vi "Associated Power Technologies 8500 Series Step Mode.vi"() -> ()   [LabVIEW 2014]
doc: "This VI is an example for controlling the power source, APT-8500 series, of Associated Power Technologies. \n\nThis vi shows how to configure and control the APT8500 series in step mode."
uses:
  <instrlib>/Associated Power Technologies 8500 Series/Public/Configure/Step Mode/Step Mode - Add File.vi
  <instrlib>/Associated Power Technologies 8500 Series/Public/Configure/Step Mode/Step Mode - Edit File.vi
  <instrlib>/Associated Power Technologies 8500 Series/Public/Configure/Step Mode/Step Mode - Configure Step Count.vi
  <instrlib>/Associated Power Technologies 8500 Series/Public/Configure/Step Mode/Step Mode - Configure Trigger Source.vi
  <instrlib>/Associated Power Technologies 8500 Series/Public/Configure/Step Mode/Step Mode - Configure Base.vi
  <instrlib>/Associated Power Technologies 8500 Series/Public/Configure/Step Mode/Step Mode - Configure Range.vi
  <instrlib>/Associated Power Technologies 8500 Series/Public/Configure/Step Mode/Step Mode - Configure Output Waveform.vi
  <instrlib>/Associated Power Technologies 8500 Series/Public/Configure/Step Mode/Step Mode - Configure Start Angle.vi
  <instrlib>/Associated Power Technologies 8500 Series/Public/Configure/Step Mode/Step Mode - Configure AC Voltage.vi
  <instrlib>/Associated Power Technologies 8500 Series/Public/Configure/Step Mode/Step Mode - Configure Frequency.vi
  <instrlib>/Associated Power Technologies 8500 Series/Public/Configure/Step Mode/Step Mode - Configure DC Voltage.vi
  <instrlib>/Associated Power Technologies 8500 Series/Public/Configure/Step Mode/Step Mode - Configure delta AC Voltage.vi
  <instrlib>/Associated Power Technologies 8500 Series/Public/Configure/Step Mode/Step Mode - Configure delta Frequency.vi
  <instrlib>/Associated Power Technologies 8500 Series/Public/Configure/Step Mode/Step Mode - Configure delta DC Voltage.vi
  <instrlib>/Associated Power Technologies 8500 Series/Public/Configure/Step Mode/Step Mode - Configure Cycle.vi
  <instrlib>/Associated Power Technologies 8500 Series/Public/Configure/Step Mode/Step Mode - Configure Time Unit.vi
  <instrlib>/Associated Power Technologies 8500 Series/Public/Configure/Step Mode/Step Mode - Configure Dwell Time.vi
  <instrlib>/Associated Power Technologies 8500 Series/Public/Configure/Step Mode/Step Mode - Configure THD.vi
  <instrlib>/Associated Power Technologies 8500 Series/Public/Configure/Step Mode/Step Mode - Load File.vi
  <instrlib>/Associated Power Technologies 8500 Series/Public/Data/Measurement/Read All Measurements.vi
  <instrlib>/Associated Power Technologies 8500 Series/Associated Power Technologies 8500 Series.lvlib
panel:
  out "All Measurements":T1
  in  "Stop":bool
  in  "Step Mode Configurations":T2={"Step Count"=5, "Trigger Source"=0, "Base"=0, "Range"=0, "Waveform Type"=0, "Start Angle"=90, "AC Voltage"=50.0, "Frequency"=60.0, "DC Voltage"=10.0, "Delta AC Voltage"=20.0, "Delta Frequency"=10.0, "Delta DC Voltage"=10.0, "Unit"=1, "Dwell Time"=2.0, "Cycles"=2, "THD"=30.0} {"Step Count" max=50000; "Trigger Source" items=["AUTO", "MANUAL"]; "Base" items=["TIME", "CYCLE"]; "Range" items=["AUTO", "HIGH", "LOW"]; "Waveform Type" items=["Sine", "Triangle", "Square", "Clipped"]; "Start Angle" max=359; "AC Voltage" min=0.0 max=310.0; "Frequency" min=5.0 max=1200.0; "DC Voltage" min=0.0 max=420.0; "Delta AC Voltage" min=0.0 max=310.0; "Delta Frequency" min=0.0 max=1200.0; "Delta DC Voltage" min=0.0 max=420.0; "Unit" items=["MS", "SECOND", "MINUTE", "HOUR"]; "Dwell Time" min=1.0 max=999.9 step=0.1; "Cycles" max=50000; "THD" min=0.0 max=46.0 step=0.1}
  in  "Serial Configuration":T3={"Baud Rate"=115200, "Parity"=0, "Data Bits"=8, "Stop Bits"=10, "Flow Control"=0} {"Flow Control" items=["None", "XON/XOFF", "RTS/CTS", "XON/XOFF & RTS/CTS", "DTR/DSR", "XON/XOFF & DTR/DSR"]; "Stop Bits" items=["1.0"=10, "1.5"=15, "2.0"=20]; "Data Bits" items=["7"=7, "8"=8]; "Parity" items=["None", "Odd", "Even", "Mark", "Space"]; "Baud Rate" items=["300"=300, "600"=600, "1200"=1200, "2400"=2400, "4800"=4800, "9600"=9600, "19200"=19200, "38400"=38400, "115200"=115200]}
  in  "VISA resource name":refnum<visa-resource-name>
  # "Step Mode Operation of APT-8500 Series"
  # "Initialization"
  # "Configurations"
  # "Meters"
  # "(c) 2020 Associated Power Technologies.  ALL RIGHTS RESERVED."
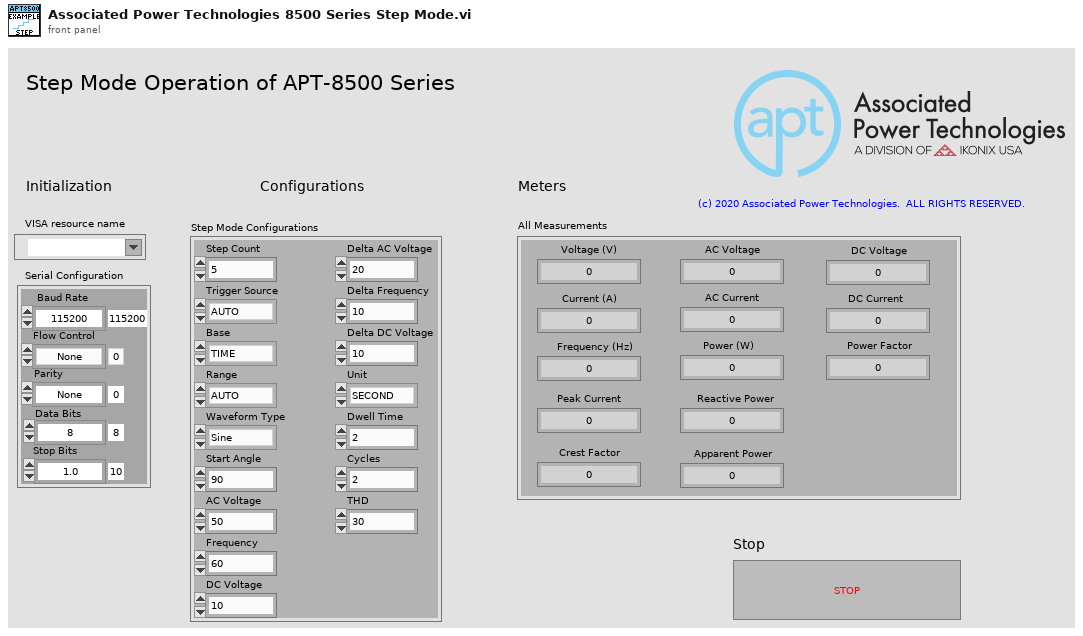
[diagram p1: front panel]
types:
  T1 = cluster{"Voltage (V)":dbl, "AC Voltage":dbl, "DC Voltage":dbl, "Current (A)":dbl, "AC Current":dbl, "DC Current":dbl, "Frequency (Hz)":dbl, "Power (W)":dbl, "Power Factor":dbl, "Peak Current":dbl, "Reactive Power":dbl, "Crest Factor":dbl, "Apparent Power":dbl}
  T2 = cluster{"Step Count":u16, "Trigger Source":u16, "Base":u16, "Range":u16, "Waveform Type":u16, "Start Angle":u16, "AC Voltage":dbl, "Frequency":dbl, "DC Voltage":dbl, "Delta AC Voltage":dbl, "Delta Frequency":dbl, "Delta DC Voltage":dbl, "Unit":u16, "Dwell Time":dbl, "Cycles":u32, "THD":dbl}
  T3 = cluster{"Baud Rate":u32, "Parity":u16, "Data Bits":u16, "Stop Bits":u16, "Flow Control":u16}
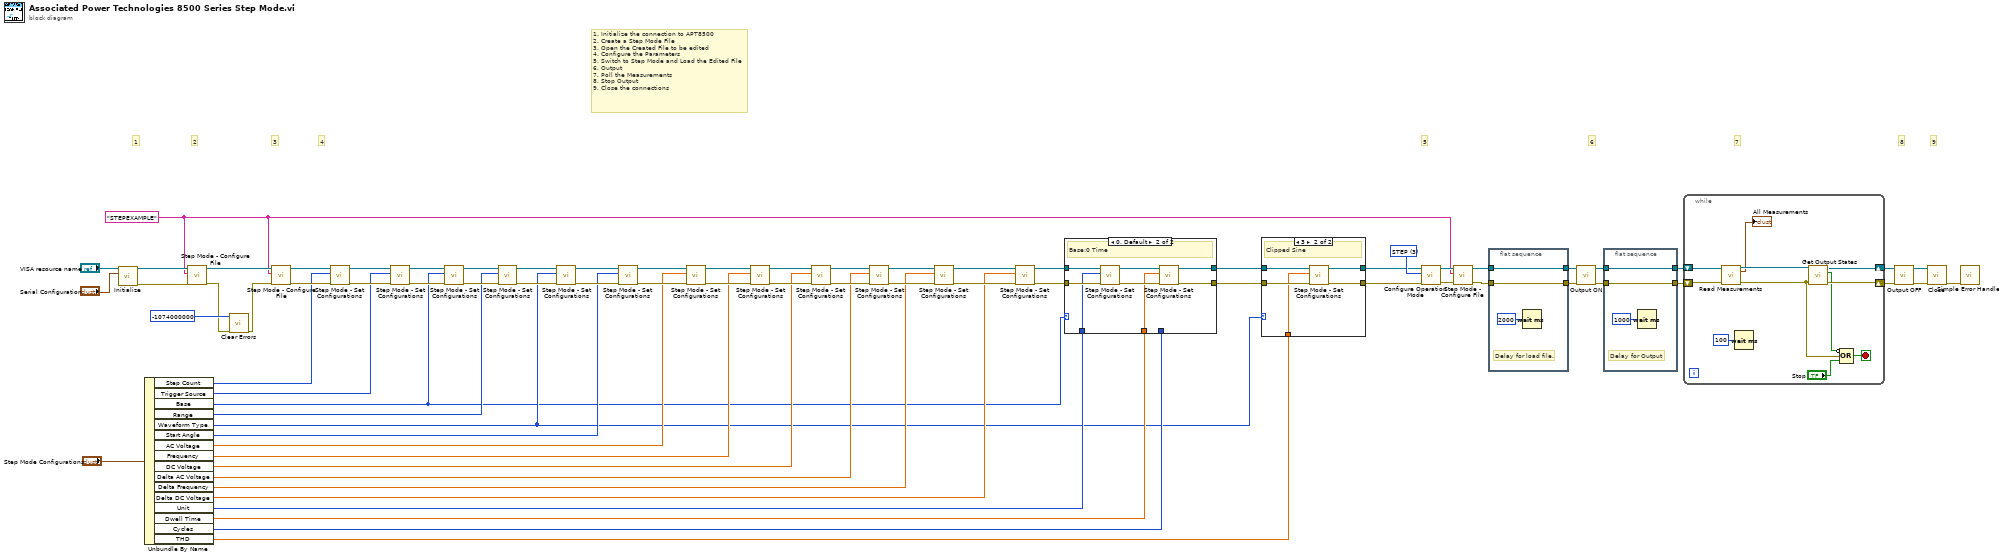
[diagram p0: block diagram]
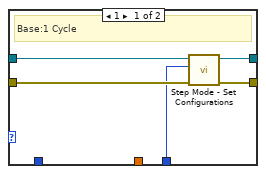
[diagram p3: hidden frame]
diagram:
  w6 = "STEPEXAMPLE" ("File Name")
  w9 = u16 3 items=["MANUAL", "LIST", "PULSE", "STEP"] ("Operation Mode")
  # "1. Initialize the connection to APT8500\n2. Create a Step Mode File\n3. Open the Created File to be edited\n4. Configure the Parameters\n5. Switch to Step Mode and Load the Edited File\n6. Output\n7. Poll the Measurements\n8. Stop Output\n9. Close the connections"
  # "9"
  # "8"
  # "7"
  # "6"
  # "5"
  # "4"
  # "3"
  # "2"
  # "1"
  n1 = call <instrlib>:"Initialize.vi"("VISA resource name"="VISA resource name", "Serial Configuration"="Serial Configuration") -> ("VISA resource name out"=w72:refnum<visa-resource-name>, "error out"=w71:errorcluster)  [unwired: 12 in]
  n2 = Unbundle By Name("Step Mode Configurations") -> ("Step Count"=w35:u16, "Trigger Source"=w34:u16, "Base"=w5:u16, "Range"=w33:u16, "Waveform Type"=w21:u16, "Start Angle"=w32:u16, "AC Voltage"=w31:dbl, "Frequency"=w30:dbl, "DC Voltage"=w29:dbl, "Delta AC Voltage"=w28:dbl, "Delta Frequency"=w27:dbl, "Delta DC Voltage"=w26:dbl, "Unit"=w25:u16, "Dwell Time"=w24:dbl, "Cycles"=w23:u32, "THD"=w22:dbl)
  n3 = call-poly <instrlib>:"Step Mode - Configure File.vi"("error in (no error)"=w71, "File Name"=w6, "VISA resource name"=w72) -> ("error out"=w66:errorcluster, "VISA resource name out"=w68:refnum<visa-resource-name>)  [unwired: 7 in]
  n4 = call <vilib>:"Clear Errors.vi"("error in (no error)"=w66, "specific error code to clear (0: all)"=-1074000000) -> ("error out"=w65:errorcluster)  [unwired: 4 in, 1 out]
  n5 = call-poly <instrlib>:"Step Mode - Configure File.vi"("error in (no error)"=w65, "File Name"=w6, "VISA resource name"=w68) -> ("error out"=w63:errorcluster, "VISA resource name out"=w64:refnum<visa-resource-name>)  [unwired: 7 in]
  n6 = call-poly <instrlib>:"Step Mode - Set Configurations.vi"("error in (no error)"=w63, "Step Count"=w35, "VISA resource name"=w64) -> ("error out"=w61:errorcluster, "VISA resource name out"=w62:refnum<visa-resource-name>)  [unwired: 7 in]
  n7 = call-poly <instrlib>:"Step Mode - Set Configurations.vi"("error in (no error)"=w61, "Trigger Source"=w34, "VISA resource name"=w62) -> ("error out"=w59:errorcluster, "VISA resource name out"=w60:refnum<visa-resource-name>)  [unwired: 7 in]
  n8 = call-poly <instrlib>:"Step Mode - Set Configurations.vi"("error in (no error)"=w59, "Base"=w5, "VISA resource name"=w60) -> ("error out"=w57:errorcluster, "VISA resource name out"=w58:refnum<visa-resource-name>)  [unwired: 7 in]
  n9 = call-poly <instrlib>:"Step Mode - Set Configurations.vi"("error in (no error)"=w57, "Range"=w33, "VISA resource name"=w58) -> ("error out"=w55:errorcluster, "VISA resource name out"=w56:refnum<visa-resource-name>)  [unwired: 7 in]
  n10 = call-poly <instrlib>:"Step Mode - Set Configurations.vi"("error in (no error)"=w55, "Waveform Type"=w21, "VISA resource name"=w56) -> ("error out"=w54:errorcluster, "VISA resource name out"=w53:refnum<visa-resource-name>)  [unwired: 7 in]
  n11 = call-poly <instrlib>:"Step Mode - Set Configurations.vi"("error in (no error)"=w54, "Start Angle(degree)"=w32, "VISA resource name"=w53) -> ("error out"=w51:errorcluster, "VISA resource name out"=w52:refnum<visa-resource-name>)  [unwired: 7 in]
  n12 = call-poly <instrlib>:"Step Mode - Set Configurations.vi"("error in (no error)"=w51, "AC Voltage"=w31, "VISA resource name"=w52) -> ("error out"=w50:errorcluster, "VISA resource name out"=w49:refnum<visa-resource-name>)  [unwired: 7 in]
  n13 = call-poly <instrlib>:"Step Mode - Set Configurations.vi"("error in (no error)"=w50, "Frequency (60)"=w30, "VISA resource name"=w49) -> ("error out"=w47:errorcluster, "VISA resource name out"=w48:refnum<visa-resource-name>)  [unwired: 7 in]
  n14 = call-poly <instrlib>:"Step Mode - Set Configurations.vi"("error in (no error)"=w47, "DC Voltage"=w29, "VISA resource name"=w48) -> ("error out"=w45:errorcluster, "VISA resource name out"=w46:refnum<visa-resource-name>)  [unwired: 7 in]
  n15 = call-poly <instrlib>:"Step Mode - Set Configurations.vi"("error in (no error)"=w45, "Delta AC Voltage"=w28, "VISA resource name"=w46) -> ("error out"=w44:errorcluster, "VISA resource name out"=w43:refnum<visa-resource-name>)  [unwired: 7 in]
  n16 = call-poly <instrlib>:"Step Mode - Set Configurations.vi"("error in (no error)"=w44, "Delta Frequency"=w27, "VISA resource name"=w43) -> ("error out"=w41:errorcluster, "VISA resource name out"=w42:refnum<visa-resource-name>)  [unwired: 7 in]
  n17 = call-poly <instrlib>:"Step Mode - Set Configurations.vi"("error in (no error)"=w41, "Delta DC Voltage"=w26, "VISA resource name"=w42) -> ("error out"=w39:errorcluster, "VISA resource name out"=w40:refnum<visa-resource-name>)  [unwired: 7 in]
  n18 = case shown="0, Default" w5 {
    tunnel: w40 -> [w77 w85]
    tunnel: w39 -> [w76 w84]
    tunnel: [w75 w81] -> w38
    tunnel: [w74 w80] -> w37
    tunnel: w25 -> [_ w79]
    tunnel: w24 -> [_ w78]
    tunnel: w23 -> [w73 _]
    frame 1 {
      # "Base:1 Cycle"
      n19 = call-poly <instrlib>:"Step Mode - Set Configurations.vi"("error in (no error)"=w76, "Cycles"=w73, "VISA resource name"=w77) -> ("error out"=w74:errorcluster, "VISA resource name out"=w75:refnum<visa-resource-name>)  [unwired: 7 in]
    }
    frame 0, Default {
      # "Base:0 Time"
      n20 = call-poly <instrlib>:"Step Mode - Set Configurations.vi"("error in (no error)"=w84, "Unit"=w79, "VISA resource name"=w85) -> ("error out"=w82:errorcluster, "VISA resource name out"=w83:refnum<visa-resource-name>)  [unwired: 7 in]
      n21 = call-poly <instrlib>:"Step Mode - Set Configurations.vi"("error in (no error)"=w82, "Dwell Time"=w78, "VISA resource name"=w83) -> ("error out"=w80:errorcluster, "VISA resource name out"=w81:refnum<visa-resource-name>)  [unwired: 7 in]
    }
  }
  n22 = case shown="3" w21 {
    tunnel: w38 -> [w87 w92]
    tunnel: w37 -> [w86 w91]
    tunnel: w22 -> [_ w90]
    tunnel: [w87 w89] -> w8
    tunnel: [w86 w88] -> w7
    frame 0, Default {
    }
    frame 3 {
      # "Clipped Sine"
      n23 = call-poly <instrlib>:"Step Mode - Set Configurations.vi"("error in (no error)"=w91, "THD"=w90, "VISA resource name"=w92) -> ("error out"=w88:errorcluster, "VISA resource name out"=w89:refnum<visa-resource-name>)  [unwired: 7 in]
    }
  }
  n24 = call <instrlib>:"Configure Operation Mode.vi"("error in (no error)"=w7, "Operation Mode (MANUAL)"=w9, "VISA resource name"=w8) -> ("error out"=w10:errorcluster, "VISA resource name out"=w11:refnum<visa-resource-name>)  [unwired: 7 in]
  n25 = call-poly <instrlib>:"Step Mode - Configure File.vi"("error in (no error)"=w10, "File Name"=w6, "VISA resource name"=w11) -> ("error out"=w13:errorcluster, "VISA resource name out"=w15:refnum<visa-resource-name>)  [unwired: 7 in]
  n26 = flat-sequence {
    tunnel: [w95] -> w16
    tunnel: w15 -> [w95]
    tunnel: [w94] -> w14
    tunnel: w13 -> [w94]
    frame #0 {
      # "Delay for load file."
      n27 = Wait (ms)(milliseconds to wait=u32 2000) -> ()  [unwired: 1 out]
    }
  }
  n28 = call <instrlib>:"Output ON.vi"("VISA resource name"=w16, "error in (no error)"=w14) -> ("VISA resource name out"=w1:refnum<visa-resource-name>, "error out"=w3:errorcluster)  [unwired: 12 in]
  n29 = flat-sequence {
    tunnel: [w97] -> w4
    tunnel: w3 -> [w97]
    tunnel: [w96] -> w2
    tunnel: w1 -> [w96]
    frame #0 {
      # "Delay for Output"
      n30 = Wait (ms)(milliseconds to wait=u32 1000) -> ()  [unwired: 1 out]
    }
  }
  n31 = while {
    shift-right: [w103] -> w19
    shift-left: w2 -> [w107]
    shift-right: [w101] -> w20
    shift-left: w4 -> [w106]
    stop <- w109 stop-if-true
    n32 = call-poly <instrlib>:"Read Measurements.vi"("VISA resource name"=w107, "error in (no error)"=w106) -> ("VISA resource name out"=w104:refnum<visa-resource-name>, "All Measurements"=→"All Measurements":T1, "error out"=w102:errorcluster)  [unwired: 11 in]
    n33 = Wait (ms)(milliseconds to wait=u32 100) -> ()  [unwired: 1 out]
    n34 = call <instrlib>:"Get Output States.vi"("error in (no error)"=w102, "VISA resource name"=w104) -> ("error out"=w101:errorcluster, "Output?"=w100:bool, "VISA resource name out"=w103:refnum<visa-resource-name>)  [unwired: 7 in]
    n35 = Compound Arithmetic op=OR(invert w100, w102, "Stop") -> (w109:bool)
  }
  n36 = call <instrlib>:"Output OFF.vi"("VISA resource name"=w19, "error in (no error)"=w20) -> ("VISA resource name out"=w18:refnum<visa-resource-name>, "error out"=w17:errorcluster)  [unwired: 12 in]
  n37 = call <instrlib>:"Close.vi"("VISA resource name"=w18, "error in (no error)"=w17) -> ("error out"=w12:errorcluster)  [unwired: 13 in]
  n38 = call <vilib>:"Simple Error Handler.vi"("error in (no error)"=w12) -> ()  [unwired: 4 in, 5 out]
